vi "Waveform Generator.vi"(0 "Exposure /ms":dbl=10.0 format="%0.2p", 1 "FOV max / V":dbl=10.0 format="%0.2p", 2 "Samples per ms":dbl=10.0 format="%0.2p", 3 "Relax /ms":dbl=10.0 format="%0.2p", 4 "FOV min/ V":dbl=10.0 format="%0.2p") -> ()   [LabVIEW 2014]
uses:
  <vilib>/Analysis/1siggen.llb/Ramp Pattern by Samples.vi
  <vilib>/Analysis/NI_AALBase.lvlib
panel:
  out "subarray":dbl[](array[numeric])
  out "appended array":dbl[][][](array[numeric])
  out "2D":dbl[][](graph)
  in  "Z Correction Max":dbl=10.0 format="%0.2p"
  in  "Z Correction Min":dbl=10.0 format="%0.2p"
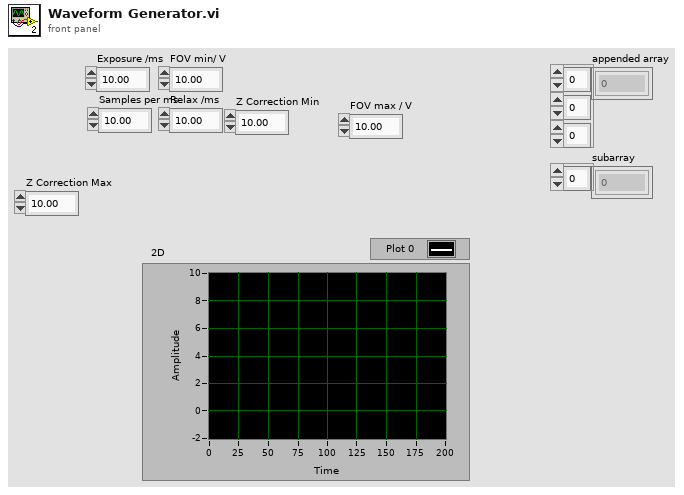
[diagram p1: front panel]
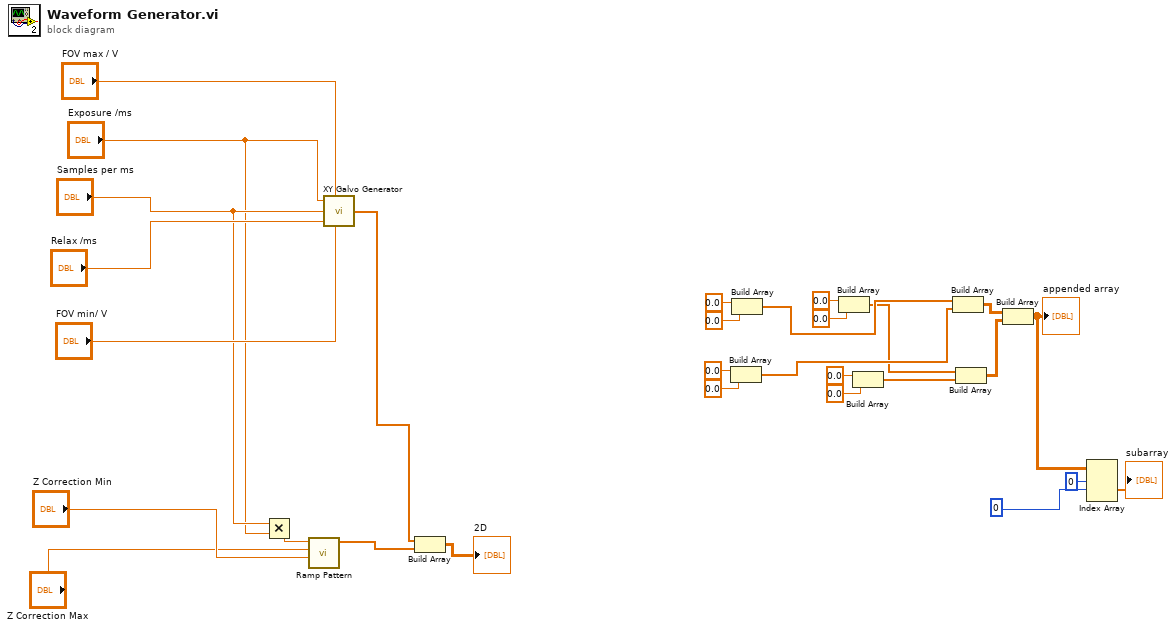
[diagram p0: block diagram]
diagram:
  n1 = Multiply(x="Samples per ms", y="Exposure /ms") -> (x*y=w22:dbl)
  n2 = call-poly <vilib>:"Ramp Pattern.vi"("start"="Z Correction Min", "end"="Z Correction Max", "samples"=w22) -> ("Ramp Pattern"=w19:dbl[])  [unwired: 7 in, 1 out]
  n3 = call "XY Galvo Generator.vi"("Exposure /ms"="Exposure /ms", "FOV max / V"="FOV max / V", "Samples per ms"="Samples per ms", "Relax /ms"="Relax /ms", "FOV min/ V"="FOV min/ V") -> ("Signal"=w20:dbl[])
  n4 = Build Array(w20, w19) -> (→"2D":dbl[][])
  n5 = Build Array(0.0 ("element"), 0.0 ("element")) -> (w9:dbl[])
  n6 = Build Array(0.0 ("element"), 0.0 ("element")) -> (w10:dbl[])
  n7 = Build Array(0.0 ("element"), 0.0 ("element")) -> (w8:dbl[])
  n8 = Build Array(0.0 ("element"), 0.0 ("element")) -> (w7:dbl[])
  n9 = Build Array(w10, w9) -> (w6:dbl[][])
  n10 = Build Array(w8, w7) -> (w5:dbl[][])
  n11 = Build Array(w6, w5) -> (w4:dbl[][][])
  "appended array" <- w4
  n12 = Index Array(array=w4, index (dim 0)=0 ("index (page)"), index (dim 1)=0 ("disabled index (row)")) -> (element=→"subarray":dbl[])  [unwired: 1 in]
